vi "child define test.vi"   [LabVIEW 2013, in "Unit Tests for Runner.lvclass"]
uses:
  Unit Tests for Runner.lvclass
  classes/Test/Test.lvclass
  classes/Assert/Assert.lvclass
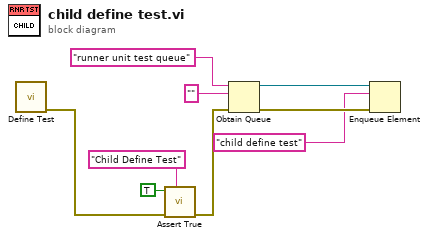
[diagram p0: block diagram]
diagram:
  n1 = call "Define Test.vi"() -> ("error out"=w2:errorcluster)  [unwired: 11 in]
  n2 = call "Assert True.vi"("Label"="Child Define Test", "error in (no error)"=w2, "True?"=TRUE) -> ("error out"=w1:errorcluster)  [unwired: 8 in]
  n3 = Obtain Queue(name (unnamed)="runner unit test queue", element data type="", error in (no error)=w1) -> (queue out=w7:refnum<queue>, error out=w6:errorcluster)  [unwired: 2 in, 1 out]
  n4 = Enqueue Element(queue=w7, element="child define test", error in (no error)=w6) -> ()  [unwired: 1 in, 3 out]
